vi "Write load bitfile.vi"(8 "error in":errorcluster, 10 "load bitfile":bool, 11 "PL_Target Configuration in":refnum<class "PL_Target Configuration.lvclass">) -> (0 "error out":errorcluster, 3 "PL_Target Configuration out":refnum<class "PL_Target Configuration.lvclass">)   [LabVIEW 2013, in "PL_Target Configuration.lvclass"]
uses:
  PL_Target Configuration.lvclass
  PL_Target Configuration.lvclass/PL_Target Configuration.ctl
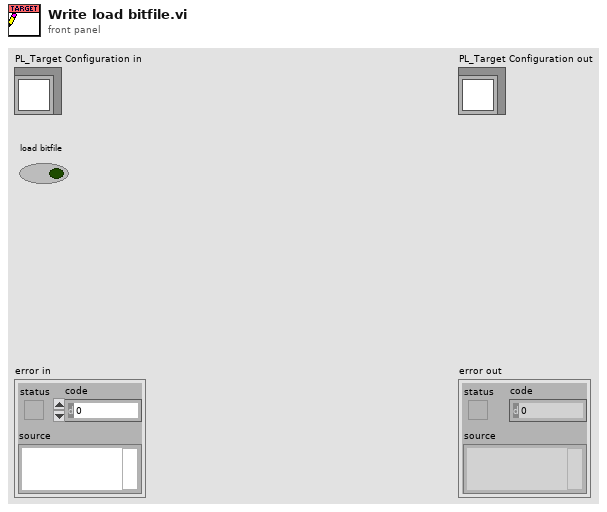
[diagram p1: front panel]
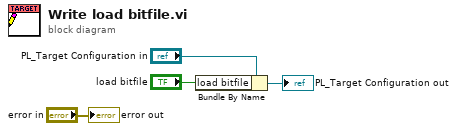
[diagram p0: block diagram]
diagram:
  n1 = Bundle By Name(cluster="PL_Target Configuration in", "load bitfile"="load bitfile") -> (→"PL_Target Configuration out":refnum<class "PL_Target Configuration.lvclass">)
  "error out" <- "error in"
